vi "Scripting_FindNodeOnDiagram.vi"(0 "ViRef(Ignored If Not Wired)":refnum<vi>, 1 "NodeTypesToSearchFor":string[](array[string]), 2 "Diagram(Ignored If Not Wired)":refnum<vi>, 5 "error in (no error)":errorcluster) -> (15 "Nodes":refnum<vi>[](array[refnum]), 19 "error out":errorcluster)   [LabVIEW 2012]
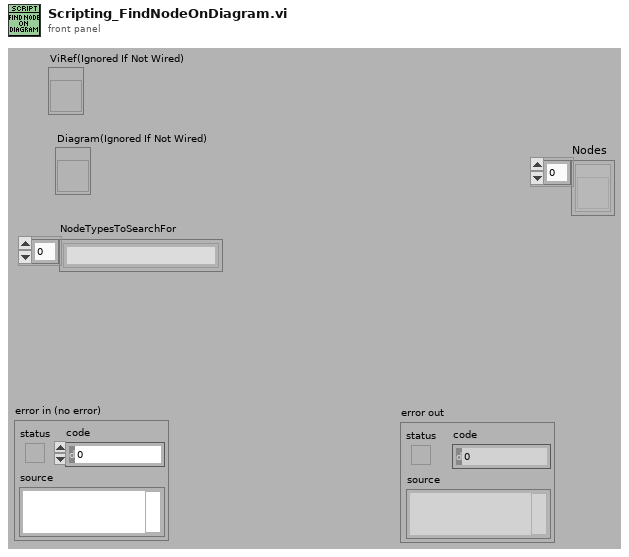
[diagram p1: front panel]
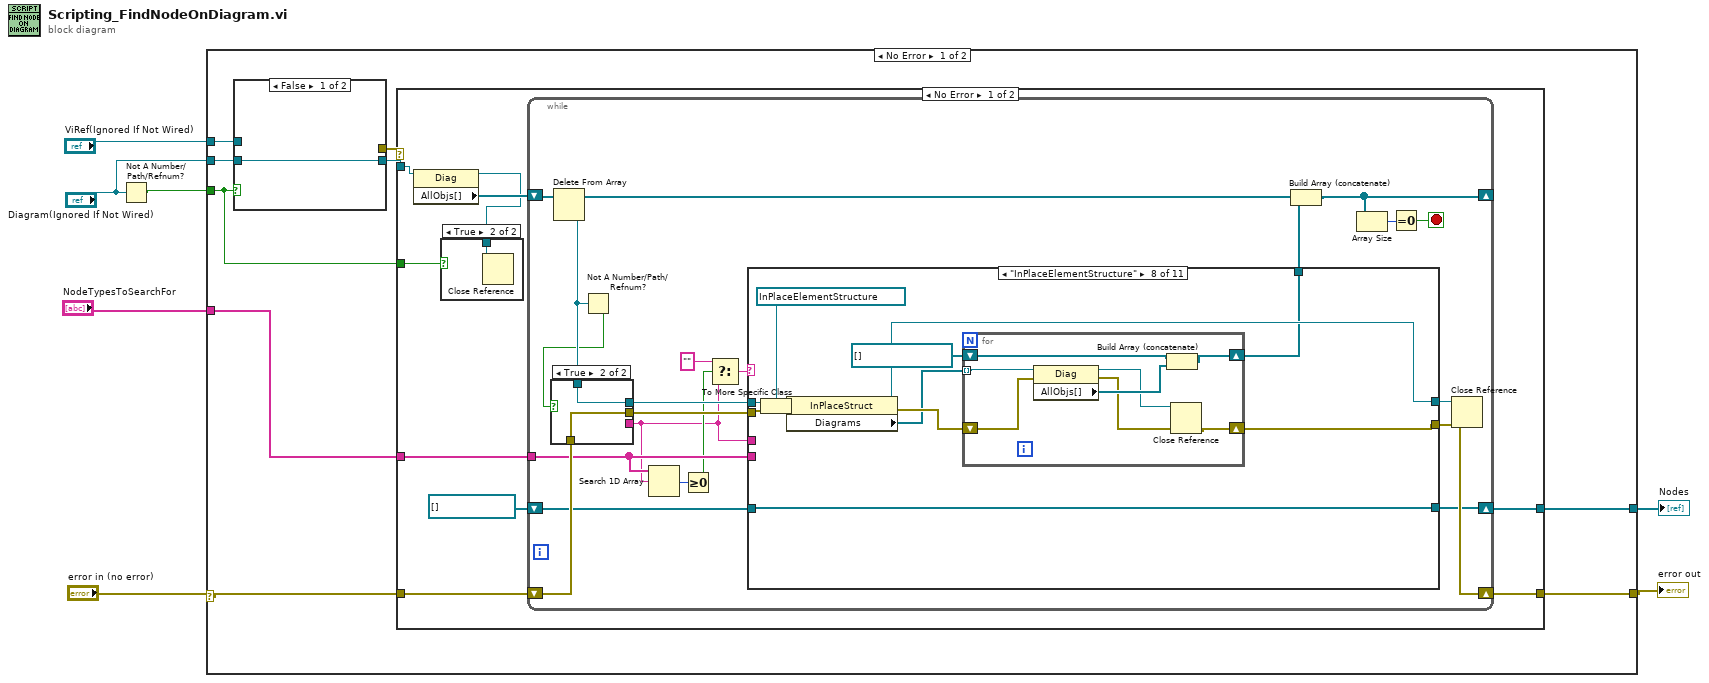
[diagram p0: block diagram]
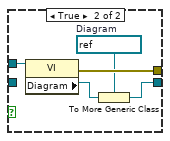
[diagram p2: hidden frame]
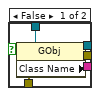
[diagram p4: hidden frame]
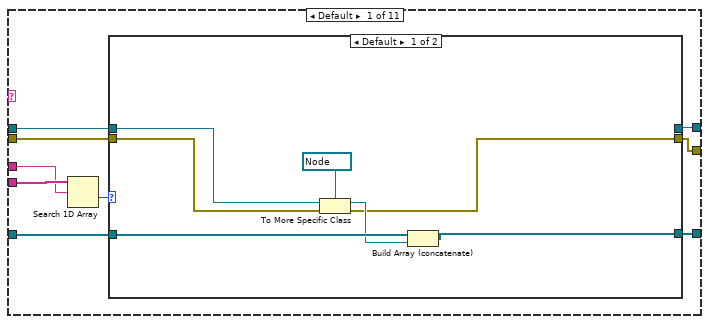
[diagram p5: hidden frame]
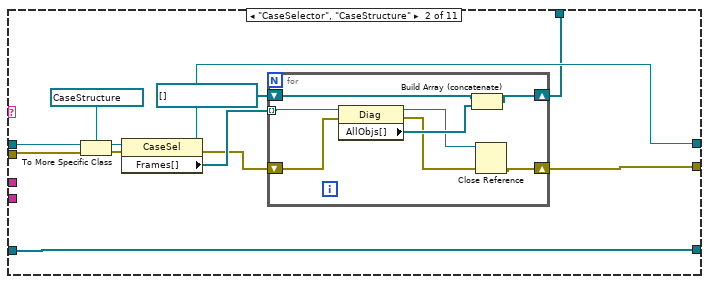
[diagram p7: hidden frame]
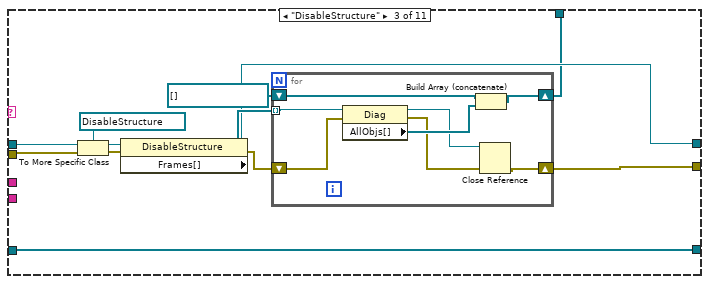
[diagram p8: hidden frame]
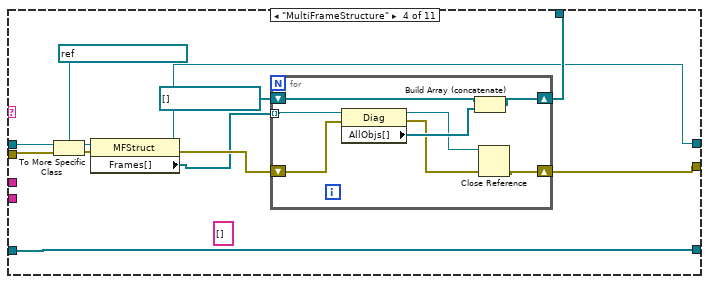
[diagram p9: hidden frame]
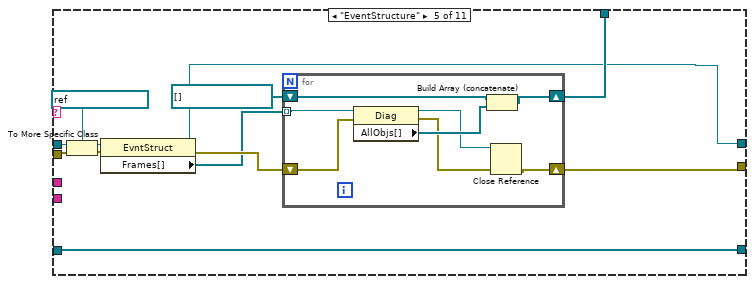
[diagram p10: hidden frame]
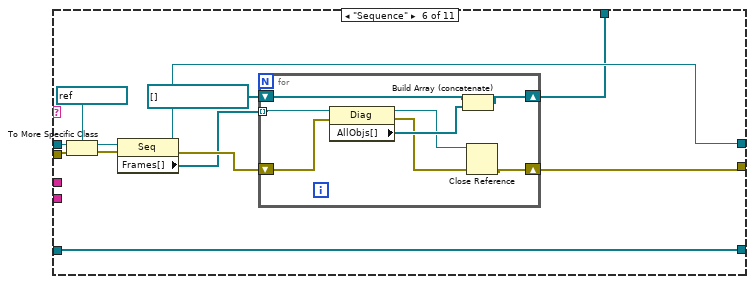
[diagram p11: hidden frame]
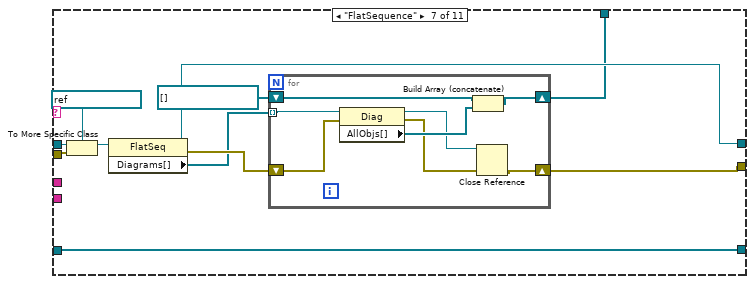
[diagram p12: hidden frame]
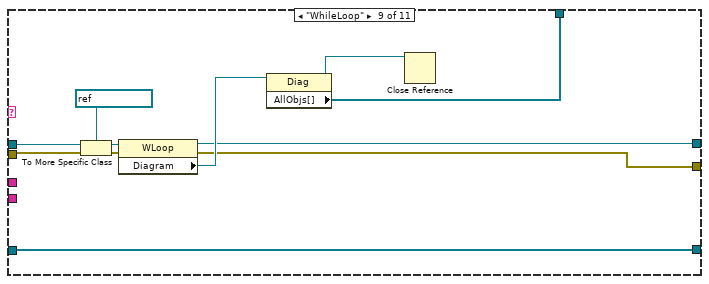
[diagram p13: hidden frame]
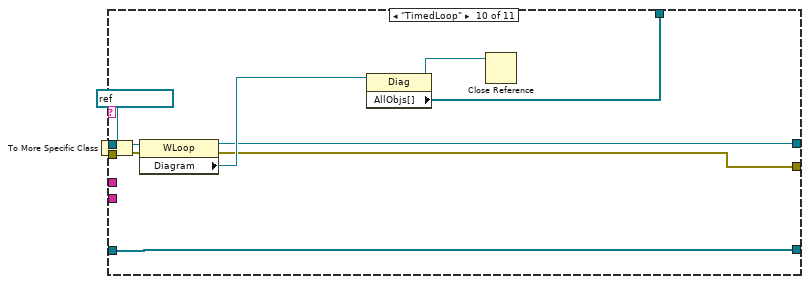
[diagram p14: hidden frame]
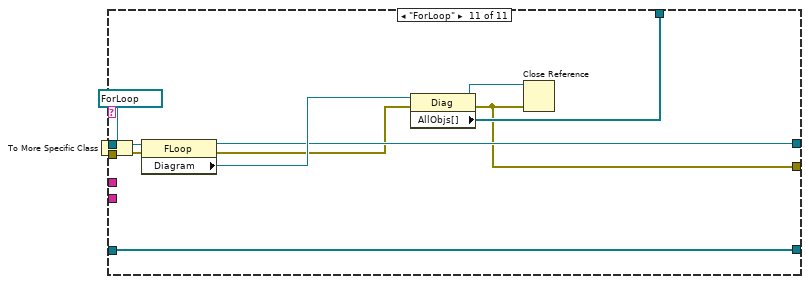
[diagram p15: hidden frame]
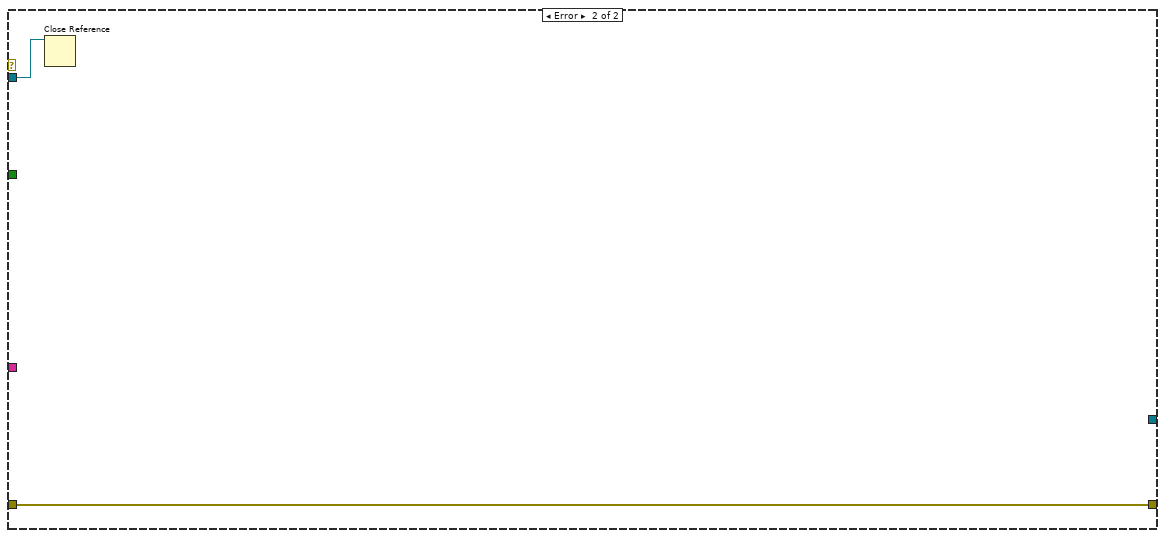
[diagram p16: hidden frame]
diagram:
  n1 = Not A Number/Path/Refnum?(number/path/refnum="Diagram(Ignored If Not Wired)") -> (NaN/Path/Refnum?=w2:bool)
  n2 = case shown="No Error" "error in (no error)" {
    selector: "error in (no error)" -> [w11 w254]
    tunnel: [w16 w254] -> w7
    tunnel: "NodeTypesToSearchFor" -> [w15 _]
    tunnel: "ViRef(Ignored If Not Wired)" -> [w14 _]
    tunnel: [w10 _] -> w3
    tunnel: w2 -> [w8 _]
    tunnel: "Diagram(Ignored If Not Wired)" -> [w9 _]
    frame No Error {
      n3 = case shown="False" w8 {
        tunnel: w14 -> [_ w22]
        tunnel: [w17 w18] -> w13
        tunnel: [_ w21] -> w12
        tunnel: w9 -> [w17 _]
        frame False {
        }
        frame True {
          w20 = refnum<vi> refnum  # Diagram
          n4 = property class="VI"(reference=w22) -> (error out=w21:errorcluster, "Diagram"=w19:refnum<vi>)  [unwired: 1 in, 1 out]
          n5 = To More Generic Class(target class=w20, reference=w19) -> (generic class reference=w18:refnum<vi>)
        }
      }
      n6 = case shown="No Error" w12 {
        tunnel: w13 -> [w31 w252]
        tunnel: [w29 w253] -> w16
        tunnel: w11 -> [w28 w253]
        tunnel: w15 -> [w27 _]
        tunnel: [w25 _] -> w10
        tunnel: w8 -> [w23 _]
        frame No Error {
          n7 = property class="Diag"(reference=w31) -> (reference out=w26:refnum<vi>, "AllObjs[]"=w30:refnum<vi>[])  [unwired: 1 in, 1 out]
          n8 = case shown="True" w23 {
            tunnel: w26 -> [_ w32]
            frame False {
            }
            frame True {
              n9 = Close Reference(reference=w32) -> ()  [unwired: 1 in, 1 out]
            }
          }
          n10 = while {
            shift-right: [w47] -> _
            shift-left: w30 -> [w53]
            shift-right: [w43] -> w29
            shift-left: w28 -> [w44]
            tunnel: w27 -> [w40]
            shift-right: [w41] -> w25
            shift-left: refnum<vi>[] [] ("Nodes") -> [w42]
            stop <- w51 stop-if-true
            n11 = Delete From Array(array=w53) -> (deleted portion=w34:refnum<vi>, array with subset deleted=w48:refnum<vi>[])  [unwired: 2 in]
            n12 = Not A Number/Path/Refnum?(number/path/refnum=w34) -> (NaN/Path/Refnum?=w33:bool)
            n13 = case shown="True" w33 {
              tunnel: [w58 w59] -> w50
              tunnel: [w57 w60] -> w49
              tunnel: w44 -> [w56 w59]
              tunnel: [w55 _] -> w37
              tunnel: w34 -> [w54 w60]
              frame False {
                n14 = property class="GObj"(reference=w54, error in=w56) -> (reference out=w57:refnum<vi>, error out=w58:errorcluster, "Class Name"=w55:string)
              }
              frame True {
              }
            }
            n15 = Search 1D Array(1D array=w40, element=w37) -> (index of element=w39:i32)  [unwired: 1 in]
            n16 = Greater Or Equal To 0?(x=w39) -> (x >= 0?=w38:bool)
            n17 = Select(t="", s=w38, f=w37) -> (s? t:f=w36:string)
            n18 = case shown="\"InPlaceElementStructure\"" w36 {
              tunnel: w49 -> [w68 w91 w111 w131 w151 w171 w190 w209 w228 w239 w251]
              tunnel: w50 -> [w69 w86 w106 w128 w148 w168 w189 w208 w224 w235 w247]
              tunnel: [w66 w84 w104 w121 w142 w164 w182 w202 w220 w231 w242] -> w43
              tunnel: [_ w82 w102 w123 w143 w162 w181 w201 w222 w233 w245] -> w46
              tunnel: [w67 w85 w105 w122 w141 w163 w183 w203 w221 w232 w244] -> w45
              tunnel: w40 -> [w63 _ _ _ _ _ _ _ _ _ _]
              tunnel: w42 -> [w65 w80 w100 w120 w140 w160 w180 w200 w218 w229 w240]
              tunnel: [w64 w80 w100 w120 w140 w160 w180 w200 w218 w229 w240] -> w41
              tunnel: w37 -> [w61 _ _ _ _ _ _ _ _ _ _]
              frame Default {
                n19 = Search 1D Array(1D array=w63, element=w61) -> (index of element=w62:i32)  [unwired: 1 in]
                n20 = case shown="Default" w62 {
                  tunnel: w69 -> [w70 w79]
                  tunnel: w68 -> [w72 w78]
                  tunnel: [w71 w79] -> w66
                  tunnel: [_ w78] -> w67
                  tunnel: w65 -> [w76 w77]
                  tunnel: [w75 w77] -> w64
                  frame Default {
                    n21 = To More Specific Class(target class=refnum<vi> refnum ("WhileLoop"), reference=w72, error in=w70) -> (specific class reference=w74:refnum<vi>, error out=w71:errorcluster)
                    n22 = Build Array (concatenate)(w76, w74) -> (w75:refnum<vi>[])
                  }
                  frame -1 {
                  }
                }
              }
              frame "CaseSelector", "CaseStructure" {
                n23 = To More Specific Class(target class=refnum<vi> refnum ("CaseSelector"), reference=w91, error in=w86) -> (specific class reference=w89:refnum<vi>, error out=w87:errorcluster)
                n24 = property class="CaseSel"(reference=w89, error in=w87) -> (reference out=w85:refnum<vi>, error out=w83:errorcluster, "Frames[]"=w88:refnum<vi>[])
                n25 = for {
                  tunnel: w88 -> [w99] mode=indexing
                  shift-right: [w92] -> w84
                  shift-left: w83 -> [w98]
                  shift-right: [w95] -> w82
                  shift-left: refnum<vi>[] [] -> [w97]
                  n26 = property class="Diag"(reference=w99, error in=w98) -> (reference out=w93:refnum<vi>, error out=w94:errorcluster, "AllObjs[]"=w96:refnum<vi>[])
                  n27 = Build Array (concatenate)(w97, w96) -> (w95:refnum<vi>[])
                  n28 = Close Reference(reference=w93, error in (no error)=w94) -> (error out=w92:errorcluster)
                }
              }
              frame "DisableStructure" {
                n29 = To More Specific Class(target class=refnum<vi> refnum ("CaseSelector"), reference=w111, error in=w106) -> (specific class reference=w109:refnum<vi>, error out=w107:errorcluster)
                n30 = property class="DisableStructure"(reference=w109, error in=w107) -> (reference out=w105:refnum<vi>, error out=w103:errorcluster, "Frames[]"=w108:refnum<vi>[])
                n31 = for {
                  tunnel: w108 -> [w119] mode=indexing
                  shift-right: [w112] -> w104
                  shift-left: w103 -> [w118]
                  shift-right: [w115] -> w102
                  shift-left: refnum<vi>[] [] -> [w117]
                  n32 = property class="Diag"(reference=w119, error in=w118) -> (reference out=w113:refnum<vi>, error out=w114:errorcluster, "AllObjs[]"=w116:refnum<vi>[])
                  n33 = Build Array (concatenate)(w117, w116) -> (w115:refnum<vi>[])
                  n34 = Close Reference(reference=w113, error in (no error)=w114) -> (error out=w112:errorcluster)
                }
              }
              frame "MultiFrameStructure" {
                (unwired) string[] []
                n35 = To More Specific Class(target class=refnum<vi> refnum ("MultiFrameStructure"), reference=w131, error in=w128) -> (specific class reference=w130:refnum<vi>, error out=w129:errorcluster)
                n36 = property class="MFStruct"(reference=w130, error in=w129) -> (reference out=w122:refnum<vi>, error out=w125:errorcluster, "Frames[]"=w124:refnum<vi>[])
                n37 = for {
                  tunnel: w124 -> [w139] mode=indexing
                  shift-right: [w132] -> w121
                  shift-left: w125 -> [w138]
                  shift-right: [w135] -> w123
                  shift-left: refnum<vi>[] [] -> [w137]
                  n38 = property class="Diag"(reference=w139, error in=w138) -> (reference out=w133:refnum<vi>, error out=w134:errorcluster, "AllObjs[]"=w136:refnum<vi>[])
                  n39 = Build Array (concatenate)(w137, w136) -> (w135:refnum<vi>[])
                  n40 = Close Reference(reference=w133, error in (no error)=w134) -> (error out=w132:errorcluster)
                }
              }
              frame "EventStructure" {
                n41 = To More Specific Class(target class=refnum<vi> refnum ("EventStructure"), reference=w151, error in=w148) -> (specific class reference=w150:refnum<vi>, error out=w149:errorcluster)
                n42 = property class="EvntStruct"(reference=w150, error in=w149) -> (reference out=w141:refnum<vi>, error out=w145:errorcluster, "Frames[]"=w144:refnum<vi>[])
                n43 = for {
                  tunnel: w144 -> [w159] mode=indexing
                  shift-right: [w152] -> w142
                  shift-left: w145 -> [w158]
                  shift-right: [w155] -> w143
                  shift-left: refnum<vi>[] [] -> [w157]
                  n44 = property class="Diag"(reference=w159, error in=w158) -> (reference out=w153:refnum<vi>, error out=w154:errorcluster, "AllObjs[]"=w156:refnum<vi>[])
                  n45 = Build Array (concatenate)(w157, w156) -> (w155:refnum<vi>[])
                  n46 = Close Reference(reference=w153, error in (no error)=w154) -> (error out=w152:errorcluster)
                }
              }
              frame "Sequence" {
                n47 = To More Specific Class(target class=refnum<vi> refnum ("Sequence"), reference=w171, error in=w168) -> (specific class reference=w170:refnum<vi>, error out=w169:errorcluster)
                n48 = property class="Seq"(reference=w170, error in=w169) -> (reference out=w163:refnum<vi>, error out=w165:errorcluster, "Frames[]"=w161:refnum<vi>[])
                n49 = for {
                  tunnel: w161 -> [w179] mode=indexing
                  shift-right: [w172] -> w164
                  shift-left: w165 -> [w178]
                  shift-right: [w175] -> w162
                  shift-left: refnum<vi>[] [] -> [w177]
                  n50 = property class="Diag"(reference=w179, error in=w178) -> (reference out=w173:refnum<vi>, error out=w174:errorcluster, "AllObjs[]"=w176:refnum<vi>[])
                  n51 = Build Array (concatenate)(w177, w176) -> (w175:refnum<vi>[])
                  n52 = Close Reference(reference=w173, error in (no error)=w174) -> (error out=w172:errorcluster)
                }
              }
              frame "FlatSequence" {
                n53 = To More Specific Class(target class=refnum<vi> refnum ("FlatSequence"), reference=w190, error in=w189) -> (specific class reference=w187:refnum<vi>)  [unwired: 1 out]
                n54 = property class="FlatSeq"(reference=w187) -> (reference out=w183:refnum<vi>, error out=w185:errorcluster, "Diagrams[]"=w184:refnum<vi>[])  [unwired: 1 in]
                n55 = for {
                  tunnel: w184 -> [w198] mode=indexing
                  shift-right: [w191] -> w182
                  shift-left: w185 -> [w197]
                  shift-right: [w194] -> w181
                  shift-left: refnum<vi>[] [] -> [w196]
                  n56 = property class="Diag"(reference=w198, error in=w197) -> (reference out=w192:refnum<vi>, error out=w193:errorcluster, "AllObjs[]"=w195:refnum<vi>[])
                  n57 = Build Array (concatenate)(w196, w195) -> (w194:refnum<vi>[])
                  n58 = Close Reference(reference=w192, error in (no error)=w193) -> (error out=w191:errorcluster)
                }
              }
              frame "InPlaceElementStructure" {
                n59 = To More Specific Class(target class=refnum<vi> refnum ("WhileLoop"), reference=w209, error in=w208) -> (specific class reference=w207:refnum<vi>)  [unwired: 1 out]
                n60 = property class="InPlaceStruct"(reference=w207) -> (reference out=w203:refnum<vi>, error out=w205:errorcluster, "Diagrams"=w204:refnum<vi>[])  [unwired: 1 in]
                n61 = for {
                  tunnel: w204 -> [w217] mode=indexing
                  shift-right: [w210] -> w202
                  shift-left: w205 -> [w216]
                  shift-right: [w213] -> w201
                  shift-left: refnum<vi>[] [] -> [w215]
                  n62 = property class="Diag"(reference=w217, error in=w216) -> (reference out=w211:refnum<vi>, error out=w212:errorcluster, "AllObjs[]"=w214:refnum<vi>[])
                  n63 = Build Array (concatenate)(w215, w214) -> (w213:refnum<vi>[])
                  n64 = Close Reference(reference=w211, error in (no error)=w212) -> (error out=w210:errorcluster)
                }
              }
              frame "WhileLoop" {
                n65 = To More Specific Class(target class=refnum<vi> refnum ("WhileLoop"), reference=w228, error in=w224) -> (specific class reference=w227:refnum<vi>, error out=w225:errorcluster)
                n66 = property class="WLoop"(reference=w227, error in=w225) -> (reference out=w221:refnum<vi>, error out=w220:errorcluster, "Diagram"=w223:refnum<vi>)
                n67 = property class="Diag"(reference=w223) -> (reference out=w219:refnum<vi>, "AllObjs[]"=w222:refnum<vi>[])  [unwired: 1 in, 1 out]
                n68 = Close Reference(reference=w219) -> ()  [unwired: 1 in, 1 out]
              }
              frame "TimedLoop" {
                n69 = To More Specific Class(target class=refnum<vi> refnum ("WhileLoop"), reference=w239, error in=w235) -> (specific class reference=w238:refnum<vi>, error out=w236:errorcluster)
                n70 = property class="WLoop"(reference=w238, error in=w236) -> (reference out=w232:refnum<vi>, error out=w231:errorcluster, "Diagram"=w234:refnum<vi>)
                n71 = property class="Diag"(reference=w234) -> (reference out=w230:refnum<vi>, "AllObjs[]"=w233:refnum<vi>[])  [unwired: 1 in, 1 out]
                n72 = Close Reference(reference=w230) -> ()  [unwired: 1 in, 1 out]
              }
              frame "ForLoop" {
                n73 = To More Specific Class(target class=refnum<vi> refnum ("WhileLoop"), reference=w251, error in=w247) -> (specific class reference=w250:refnum<vi>, error out=w248:errorcluster)
                n74 = property class="FLoop"(reference=w250, error in=w248) -> (reference out=w244:refnum<vi>, error out=w243:errorcluster, "Diagram"=w246:refnum<vi>)
                n75 = property class="Diag"(reference=w246, error in=w243) -> (reference out=w241:refnum<vi>, error out=w242:errorcluster, "AllObjs[]"=w245:refnum<vi>[])
                n76 = Close Reference(reference=w241, error in (no error)=w242) -> ()  [unwired: 1 out]
              }
            }
            n77 = Build Array (concatenate)(w48, w46) -> (w47:refnum<vi>[])
            n78 = Array Size(array=w47) -> (size(s)=w52:i32)
            n79 = Equal To 0?(x=w52) -> (x = 0?=w51:bool)
            n80 = Close Reference(reference=w45, error in (no error)=w43) -> ()  [unwired: 1 out]
          }
        }
        frame Error {
          n81 = Close Reference(reference=w252) -> ()  [unwired: 1 in, 1 out]
        }
      }
    }
    frame Error {
    }
  }
  "error out" <- w7
  "Nodes" <- w3
